vi "Configure Offset and Limits (Adjacent Channel Power - VBW and RBW).vi"(0 "VISA resource name":refnum<visa-resource-name>, 1 "Auto Video Bandwidth List":bool[](array[boolean])=[FALSE, FALSE, FALSE, FALSE, FALSE, FALSE], 2 "Manual Video Bandwidth Frequency List":dbl[](array[numeric])=[220000.0, 220000.0, 220000.0, 220000.0, 220000.0, 220000.0], 5 "Device Mode (1: BTS)":i32(ring)=1 items=["BTS"=1, "MS"=2], 7 "Filter Type List":i32[](array[ring])=[0, 0, 0, 0, 0, 0] items=["Gaussian", "Flattop"], 9 "Filter Bandwidth List":i32[](array[ring])=[0, 0, 0, 0, 0, 0] items=["-3dB", "-6dB"], 11 "error in (no error)":errorcluster, 12 "Auto Resolution Bandwidth List":bool[](array[boolean])=[FALSE, FALSE, FALSE, FALSE, FALSE, FALSE], 13 "Manual Resolution Bandwidth Frequency List":dbl[](array[numeric])=[120000.0, 120000.0, 120000.0, 120000.0, 120000.0, 120000.0]) -> (4 "VISA resource name out":refnum<visa-resource-name>, 15 "error out":errorcluster)   [LabVIEW 2014, in "Agilent MXA Series.lvlib"]
doc: "Configures the VBW and RBW settings under offsets and limits for ACP measurement type."
uses:
  Agilent MXA Series.lvlib
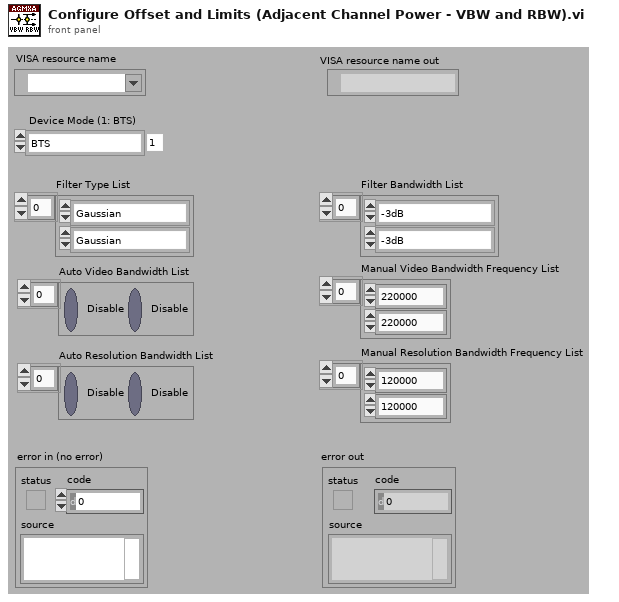
[diagram p1: front panel]
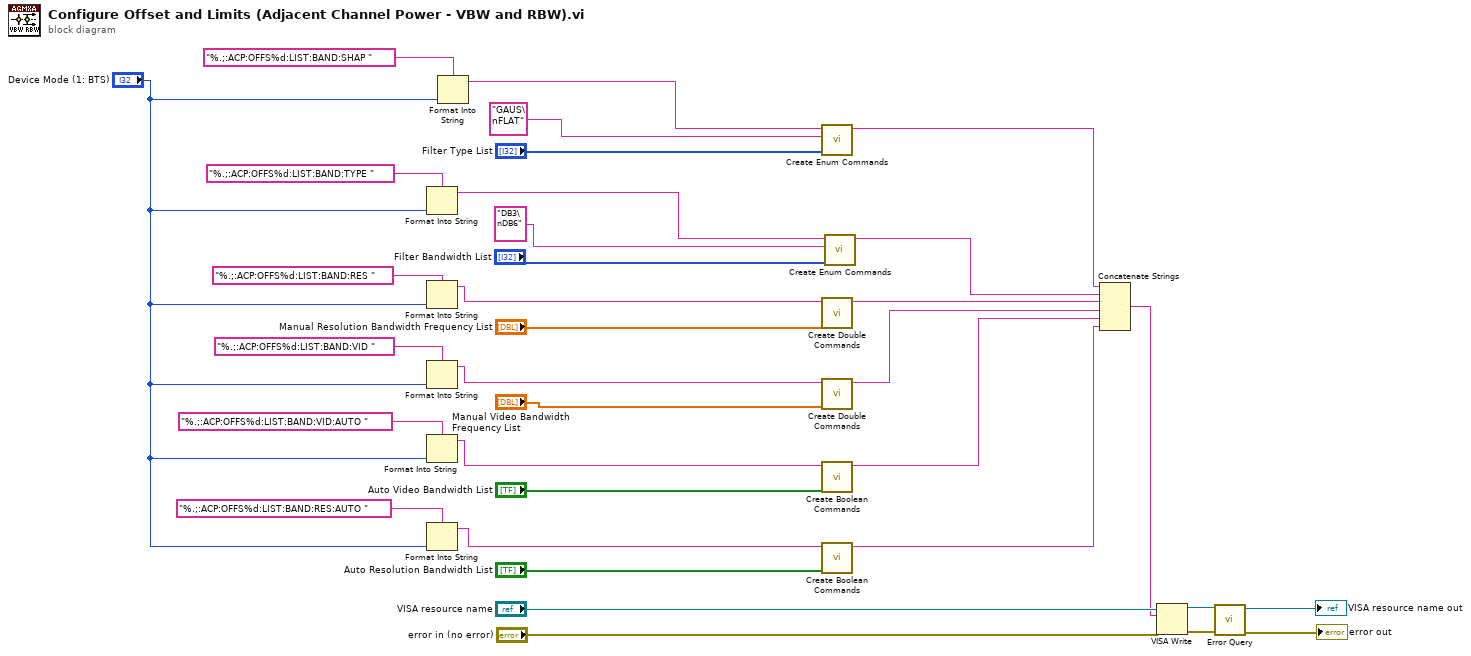
[diagram p0: block diagram]
diagram:
  n1 = Format Into String(format string="%.;:ACP:OFFS%d:LIST:BAND:TYPE ", "Device Mode (1: BTS)") -> (resulting string=w7:string)  [unwired: 2 in, 1 out]
  n2 = Format Into String(format string="%.;:ACP:OFFS%d:LIST:BAND:RES ", "Device Mode (1: BTS)") -> (resulting string=w20:string)  [unwired: 2 in, 1 out]
  n3 = Format Into String(format string="%.;:ACP:OFFS%d:LIST:BAND:VID ", "Device Mode (1: BTS)") -> (resulting string=w21:string)  [unwired: 2 in, 1 out]
  n4 = Format Into String(format string="%.;:ACP:OFFS%d:LIST:BAND:VID:AUTO ", "Device Mode (1: BTS)") -> (resulting string=w27:string)  [unwired: 2 in, 1 out]
  n5 = Format Into String(format string="%.;:ACP:OFFS%d:LIST:BAND:RES:AUTO ", "Device Mode (1: BTS)") -> (resulting string=w25:string)  [unwired: 2 in, 1 out]
  n6 = Format Into String(format string="%.;:ACP:OFFS%d:LIST:BAND:SHAP ", "Device Mode (1: BTS)") -> (resulting string=w10:string)  [unwired: 2 in, 1 out]
  n7 = call "Create Enum Commands.vi"("Enum Values"="Filter Type List", "Multi-line Text"="GAUS\nFLAT" ("format string"), "Commands"=w10) -> ("Result"=w4:string)  [unwired: 8 in]
  n8 = call "Create Double Commands.vi"("Double Values"="Manual Resolution Bandwidth Frequency List", "Commands"=w20) -> ("Result"=w2:string)  [unwired: 9 in]
  n9 = call "Create Double Commands.vi"("Double Values"="Manual Video Bandwidth Frequency List", "Commands"=w21) -> ("Result"=w13:string)  [unwired: 9 in]
  n10 = call "Create Boolean Commands.vi"("Boolean States"="Auto Video Bandwidth List", "Command"=w27) -> ("Result String"=w12:string)  [unwired: 9 in]
  n11 = call "Create Boolean Commands.vi"("Boolean States"="Auto Resolution Bandwidth List", "Command"=w25) -> ("Result String"=w11:string)  [unwired: 9 in]
  n12 = call "Create Enum Commands.vi"("Enum Values"="Filter Bandwidth List", "Multi-line Text"="DB3\nDB6" ("format string"), "Commands"=w7) -> ("Result"=w3:string)  [unwired: 8 in]
  n13 = Concatenate Strings(w4, w3, w2, w13, w12, w11) -> (w1:string)
  n14 = VISA Write(VISA resource name="VISA resource name", write buffer=w1, error in (no error)="error in (no error)") -> (VISA resource name out=w16:refnum<visa-resource-name>, error out=w17:errorcluster)  [unwired: 1 out]
  n15 = call "Error Query.vi"("error in (no error)"=w17, "VISA resource name"=w16) -> ("error out"=→"error out":errorcluster, "VISA resource name out"=→"VISA resource name out":refnum<visa-resource-name>)  [unwired: 6 in, 2 out]
